vi "Local Transition Inward.vi"(8 "error in (no error)":errorcluster, 9 "Timeout Period in ms (-1, never)":i32=-1, 10 "Target State":refnum<class "_State Machine Actor.lvclass">, 11 "_State Machine Actor in":refnum<class "_State Machine Actor.lvclass">) -> (0 "error out":errorcluster, 3 "_State Machine Actor out":refnum<class "_State Machine Actor.lvclass">)   [LabVIEW 2024]
uses:
  _State Machine Actor.lvclass/_State Machine Actor.ctl
  _State Machine Actor.lvclass
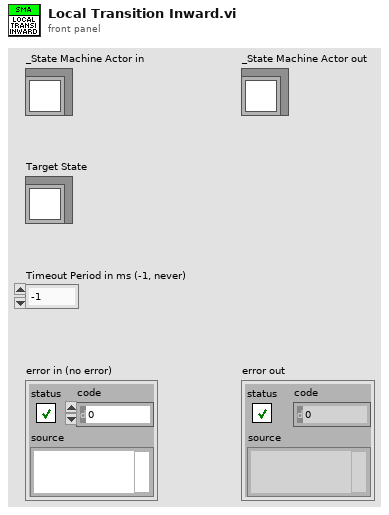
[diagram p1: front panel]
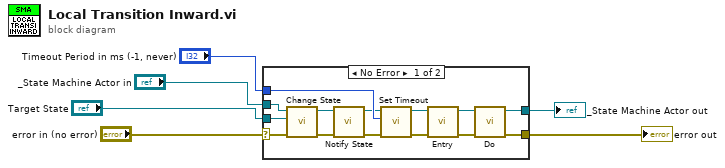
[diagram p0: block diagram]
diagram:
  n1 = case shown="No Error" "error in (no error)" {
    selector: "error in (no error)" -> [w14 w22]
    tunnel: [w13 w22] -> w5
    tunnel: [w16 w21] -> w3
    tunnel: "_State Machine Actor in" -> [w19 w21]
    tunnel: "Target State" -> [w18 _]
    tunnel: "Timeout Period in ms (-1, never)" -> [w15 _]
    frame No Error {
      n2 = call-dynamic "Change State.vi"("error in (no error)"=w14, "Target State"=w18, "_State Machine Actor in"=w19) -> ("error out"=w11:errorcluster, "_State Machine Actor out"=w12:refnum<class "_State Machine Actor.lvclass">)  [unwired: 7 in]
      n3 = call "Notify State.vi"("error in (no error)"=w11, "_State Machine Actor in"=w12) -> ("error out"=w9:errorcluster, "_State Machine Actor out"=w10:refnum<class "_State Machine Actor.lvclass">)  [unwired: 8 in]
      n4 = call "Set Timeout.vi"("error in (no error)"=w9, "Timeout Period in ms (-1, never)"=w15, "_State Machine Actor in"=w10) -> ("error out"=w20:errorcluster, "_State Machine Actor out"=w17:refnum<class "_State Machine Actor.lvclass">)  [unwired: 7 in]
      n5 = call-dynamic "Entry.vi"("error in (no error)"=w20, "State Machine Actor in"=w17) -> ("error out"=w7:errorcluster, "State Machine Actor out"=w8:refnum<class "_State Machine Actor.lvclass">)  [unwired: 8 in]
      n6 = call-dynamic "Do.vi"("error in (no error)"=w7, "_State Machine Actor in"=w8) -> ("error out"=w13:errorcluster, "_State Machine Actor out"=w16:refnum<class "_State Machine Actor.lvclass">)  [unwired: 8 in]
    }
    frame Error {
    }
  }
  "error out" <- w5
  "_State Machine Actor out" <- w3
